vi "Get Cooler Status.vi"(8 "error in (no error)":errorcluster, 11 "CCDCamera in":refnum<class "Simulated_CCD_Camera.lvclass">) -> (0 "error out":errorcluster, 3 "CCDCamera out":refnum<class "Simulated_CCD_Camera.lvclass">)   [LabVIEW 2018, in "Simulated_CCD_Camera.lvclass"]
uses:
  Simulated_CCD_Camera.lvclass
  Simulated_CCD_Camera.lvclass/Simulated_CCD_Camera.ctl
  Simulated_Cooler/Simulated_Cooler.lvclass
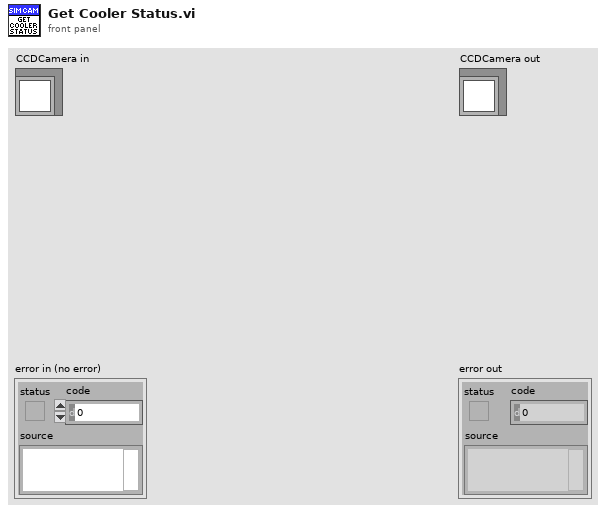
[diagram p1: front panel]
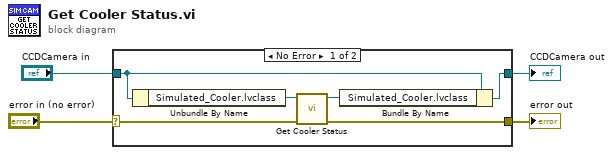
[diagram p0: block diagram]
diagram:
  n1 = case shown="No Error" "error in (no error)" {
    selector: "error in (no error)" -> [w5 w12]
    tunnel: [w6 w12] -> w3
    tunnel: [w8 w11] -> w1
    tunnel: "CCDCamera in" -> [w9 w11]
    frame No Error {
      n2 = Unbundle By Name(w9) -> ("Simulated_Cooler.lvclass"=w10:refnum<class "Simulated_Cooler.lvclass">)
      n3 = call-dynamic "Get Cooler Status.vi"("error in (no error)"=w5, "Cooler in"=w10) -> ("error out"=w6:errorcluster, "Cooler out"=w7:refnum<class "Simulated_Cooler.lvclass">)  [unwired: 8 in]
      n4 = Bundle By Name(cluster=w9, "Simulated_Cooler.lvclass"=w7) -> (w8:refnum<class "Simulated_CCD_Camera.lvclass">)
    }
    frame Error {
    }
  }
  "error out" <- w3
  "CCDCamera out" <- w1
